vi "clipconfiguration.vi"() -> ()   [LabVIEW 2009]
uses:
  <vilib>/Utility/NIReport.llb/NI_report.lvclass
  <instrlib>/Agilent 81150/Agilent 81150.lvlib
panel:
  out "XY Graph 4":cluster{"Y":dbl[], "Y":dbl[]}[][](array[cluster])
  out "XY Graph 3":cluster{"Y":dbl[], "Y":dbl[]}[][](array[cluster])
  in  "Comprobation":bool
  in  "vclip":i32[](array[numeric])=[200]
  in  "Channels init":i32[](array[numeric])=[1900]
  in  "Channels":i32[](array[numeric])=[1]
  in  "Cycles Burst":i32=10000
  out "IPR_Address":i32=23
  out "L1 Address":i32=17
  in  "L1 version":bool
  in  "Instrument VISA in":T1={"AWG VISA"="81160A", "Oscilloscope  VISA "="DSO80204B", "Integration Board IP"="172.16.7.43", "connection ID"=refnum, "report out"=refnum, "report file path"=path "D:/CTA/LevelTriggerBoardTest/TestsData/sumtrigger_delay/clipconfig"}
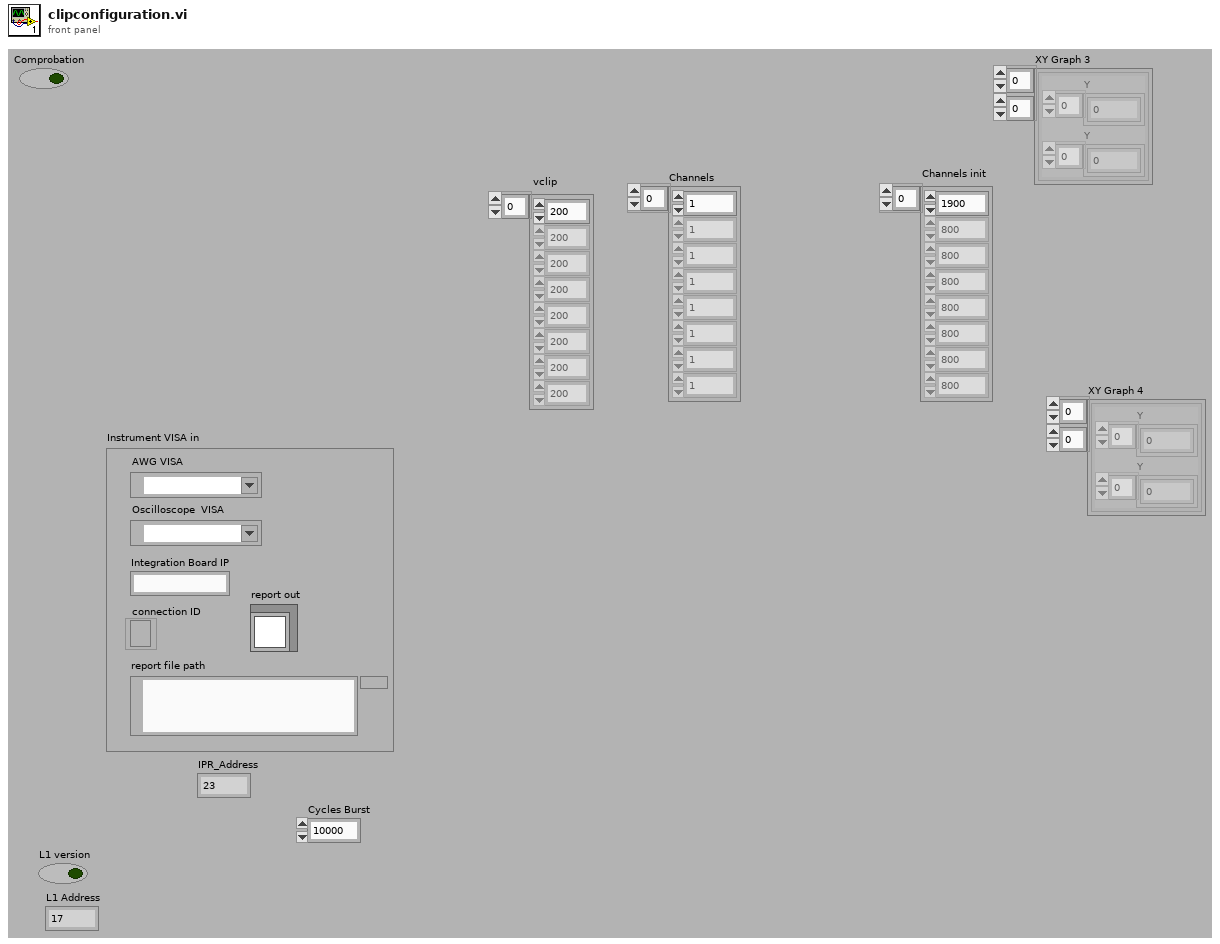
[diagram p1: front panel]
types:
  T1 = cluster{"AWG VISA":refnum<visa-resource-name>, "Oscilloscope  VISA ":refnum<visa-resource-name>, "Integration Board IP":string, "connection ID":refnum<k5>, "report out":refnum<class "NI_report.lvclass">, "report file path":path}
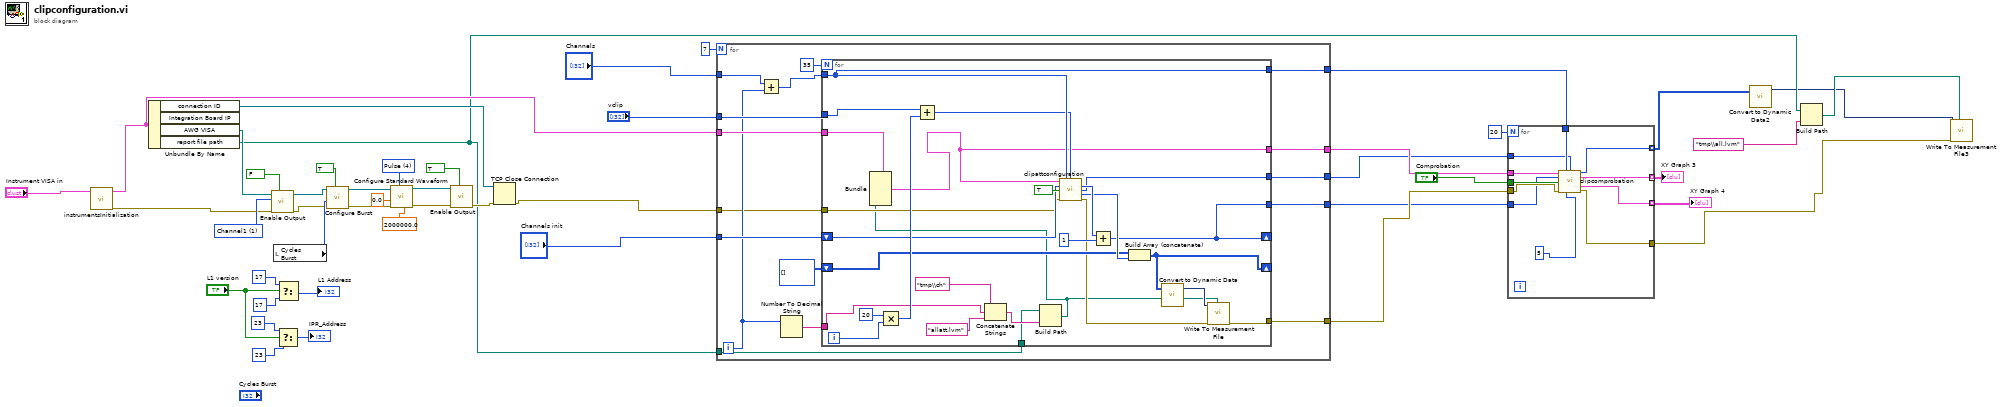
[diagram p0: block diagram]
diagram:
  (unwired) "tmp\\all.lvm" ("name or relative path")
  w39 = u16 4 items=["Sine", "Square", "Ramp Up", "Ramp Down", "Pulse", "Noise", "DC"] ("Waveform (0: Sine)")
  w45 = u16 1 items=["Channel1"=1, "Channel2"=2] ("Channel (1: Channel1)")
  n1 = call "instrumentsInitialization.vi"("Instrument VISA in"="Instrument VISA in") -> ("error out"=w23:errorcluster, "Instrument VISA out"=w19:T1)  [unwired: 9 in]
  n2 = Unbundle By Name(w19) -> ("connection ID"=w26:refnum<k5>, "AWG VISA"=w40:refnum<visa-resource-name>, "report file path"=w10:path)  [unwired: 1 out]
  n3 = call <instrlib>:"Enable Output.vi"("Enable Output (T: Enable)"=FALSE, "error in (no error)"=w23, "Channel (1: Channel1)"=w45, "VISA resource name"=w40) -> ("error out"=w25:errorcluster, "VISA resource name out"=w24:refnum<visa-resource-name>)  [unwired: 6 in]
  n4 = local read "Cycles Burst"() -> (w28:i32)
  n5 = Select(t=23 ("Address"), s="L1 version", f=23 ("Address")) -> (s? t:f=→"IPR_Address":i32)
  n6 = Select(t=17 ("Address"), s="L1 version", f=17 ("Address")) -> (s? t:f=→"L1 Address":i32)
  n7 = call <instrlib>:"Configure Burst.vi"("Enable Burst (F: Disable)"=TRUE, "error in (no error)"=w25, "Burst Count (2)"=w28, "VISA resource name"=w24) -> ("error out"=w36:errorcluster, "VISA resource name out"=w37:refnum<visa-resource-name>)  [unwired: 6 in]
  n8 = call <instrlib>:"Configure Standard Waveform.vi"("Frequency (1000.0 Hz)"=2000000.0, "Waveform (0: Sine)"=w39, "error in (no error)"=w36, "Amplitude (1.0 Vpp)"=0.0, "VISA resource name"=w37) -> ("error out"=w35:errorcluster, "VISA resource name out"=w22:refnum<visa-resource-name>)  [unwired: 5 in]
  n9 = call <instrlib>:"Enable Output.vi"("Enable Output (T: Enable)"=TRUE, "error in (no error)"=w35, "VISA resource name"=w22) -> ("error out"=w27:errorcluster)  [unwired: 7 in, 1 out]
  n10 = TCP Close Connection(connection ID=w26, error in (no error)=w27) -> (error out=w1:errorcluster)  [unwired: 1 in, 1 out]
  n11 = for {
    N: 7 -> [_]
    tunnel: "vclip" -> [w63]
    tunnel: "Channels" -> [w52]
    tunnel: w19 -> [w62]
    tunnel: "Channels init" -> [w61]
    tunnel: [w59] -> w16
    tunnel: [w58] -> w15
    tunnel: [w56] -> w12
    tunnel: w10 -> [w55]
    tunnel: [w54] -> w5
    tunnel: [w53] -> w4
    tunnel: w1 -> [w48]
    i -> [w50]
    n12 = Add(x=w52, y=w50) -> (x+y=w51:i32[])
    n13 = Number To Decimal String(number=w50) -> (decimal integer string=w49:string)  [unwired: 1 in]
    n14 = for {
      N: 35 -> [_]
      tunnel: w51 -> [w88]
      tunnel: w62 -> [w67]
      tunnel: [w65] -> w59
      tunnel: [w88] -> w58
      tunnel: w63 -> [w90]
      shift-right: [w74] -> _
      shift-left: w61 -> [w83]
      shift-right: [w78] -> _
      shift-left: i64[][] [] -> [w79]
      tunnel: [w75] -> w56
      tunnel: w55 -> [w68]
      tunnel: [w74] -> w54
      tunnel: [w73] -> w53
      tunnel: w49 -> [w70]
      tunnel: w48 -> [w66]
      i -> [w86]
      n15 = Multiply(x=20, y=w86) -> (x*y=w84:i32)
      n16 = Add(x=w90, y=w84) -> (x+y=w87:i32[])
      n17 = Concatenate Strings("tmp\\ch" ("name or relative path"), w70, "allatt.lvm" ("string")) -> (w72:string)
      n18 = Build Path(base path=w68, name or relative path=w72) -> (appended path=w64:path)
      n19 = Bundle(cluster=w67, "report file path"=w64) -> (w65:T1)  [unwired: 5 in]
      n20 = call "clipattconfiguration.vi"("input cluster"=w65, "Channels values 2"=w88, "vclip"=w87, "Channels init"=w83, "Boolean"=TRUE, "error out 2"=w66) -> ("vatt"=w81:i32[], "vclip"=w73:i32[], "appended array"=w80:i64[], "error out"=w76:errorcluster)  [unwired: 6 in]
      n21 = Add(x=w81, y=1 ("x")) -> (x+y=w74:i32[])
      n22 = Build Array (concatenate)(w79, w80) -> (w78:i64[][])
      n23 = call "Convert to Dynamic Data"("2D Array"=w78) -> ("Dynamic Data Type"=w77:dynamicdata)  [unwired: 3 in]
      n24 = call "Write To Measurement File"("Signals"=w77, "error in (no error)"=w76, "Filename"=w64) -> ("error out"=w75:errorcluster)  [unwired: 14 in, 2 out]
    }
  }
  n25 = for {
    N: 20 -> [_]
    tunnel: "Comprobation" -> [w101]
    tunnel: w16 -> [w100]
    tunnel: w12 -> [w99]
    tunnel: w15 -> [w98]
    tunnel: [w97] -> w14 mode=indexing
    tunnel: [w96] -> w13 mode=indexing
    tunnel: [w94] -> w9 mode=indexing
    tunnel: [w93] -> w7
    tunnel: w5 -> [w92]
    tunnel: w4 -> [w91]
    n26 = call "clipcomprobation.vi"("input cluster"=w100, "Channels values 2"=w98, "vclip"=w91, "Channels init"=w92, "Boolean"=w101, "error out 2"=w99, "Number points"=5 ("x")) -> ("L1  values"=w94:i32[], "XY Graph"=w97:cluster{"Y":dbl[], "Y":dbl[]}[], "XY Graph 2"=w96:cluster{"Y":dbl[], "Y":dbl[]}[], "error out"=w93:errorcluster)  [unwired: 5 in]
  }
  "XY Graph 3" <- w14
  "XY Graph 4" <- w13
  n27 = call "Convert to Dynamic Data2"("2D Array"=w9) -> ("Dynamic Data Type"=w8:dynamicdata)  [unwired: 3 in]
  n28 = Build Path(base path=w10, name or relative path="tmp\\all.lvm") -> (appended path=w11:path)
  n29 = call "Write To Measurement File3"("Signals"=w8, "error in (no error)"=w7, "Filename"=w11) -> ()  [unwired: 14 in, 3 out]
